vi "Tab_004_PH.vi"() -> ()   [LabVIEW 2021]
panel:
  out "Array 3":dbl[](array[numeric])
  in  "Array":dbl[](array[numeric])=[11.1, 14.2, 18.3, 22.4, 26.5]
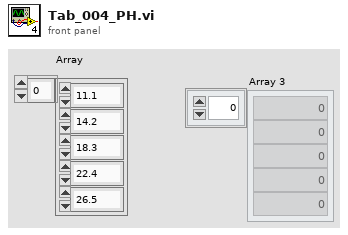
[diagram p1: front panel]
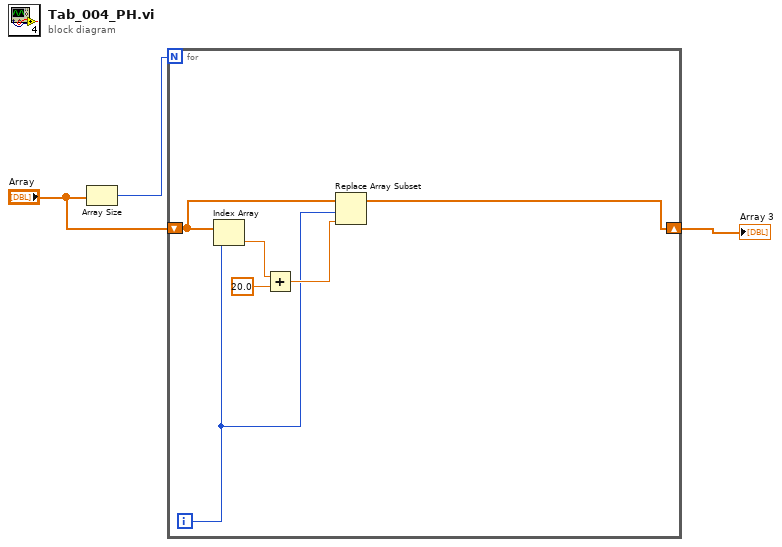
[diagram p0: block diagram]
diagram:
  n1 = Array Size(array="Array") -> (size(s)=w3:i32)
  n2 = for {
    N: w3 -> [_]
    shift-right: [w4] -> w1
    shift-left: "Array" -> [w5]
    i -> [w6]
    n3 = Index Array(array=w5, index=w6) -> (element=w8:dbl)
    n4 = Add(x=w8, y=20.0) -> (x+y=w7:dbl)
    n5 = Replace Array Subset(array=w5, new element=w7, index=w6) -> (w4:dbl[])
  }
  "Array 3" <- w1
